vi "Password_Authentication.vi"(11 "String":string) -> (1 "Access Status":string)   [LabVIEW 2017]
panel:
  out "True / False":bool=TRUE
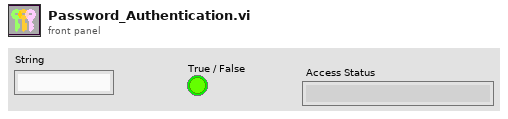
[diagram p1: front panel]
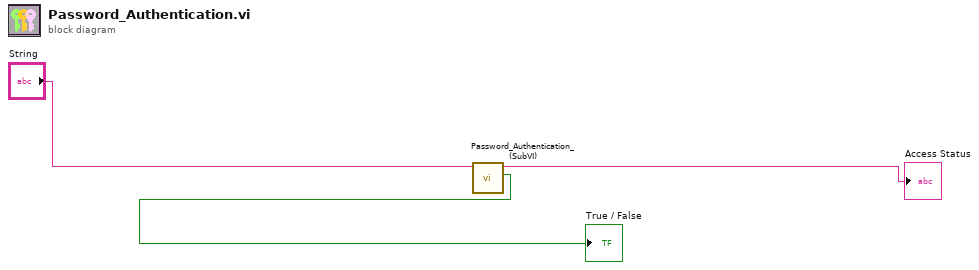
[diagram p0: block diagram]
diagram:
  n1 = call "Password_Authentication_(SubVI).vi"("String"="String") -> ("True / False"=→"True / False":bool, "Access Status"=→"Access Status":string)  [unwired: 9 in]
